vi "WCA_GET_AMC.vi"(0 "Cartridge Band":u32=10, 1 "Slave Node in":cluster{"Address":i16, "Serial Number":i8[]}={"Address"=19, "Serial Number"=[16, 71, 55, 76, 1, 8, 0, -15]} {"Serial Number" format="%.0x"; "Address" format="%.0x"}, 2 "ObjHandle in":u32, 11 "error in (no error)":errorcluster) -> (4 "ObjHandle out":u32=92930112, 8 "GET_AMC":T1={"AMC_A_DRAIN_V"=3.5023499, "AMC_A_DRAIN_C"=53.95508, "AMC_A_GATE_V"=-0.47195435, "AMC_B_DRAIN_V"=4.3559265, "AMC_B_DRAIN_C"=314.81934, "AMC_B_GATE_V"=-0.49163818, "AMC_E_DRAIN_V"=3.9920044, "AMC_E_DRAIN_C"=338.2721, "AMC_E_GATE_V"=-0.24505615, "AMC_3V_SUPPLY_V"=-13.493347, "AMC_5V_MON"=5.223694, "AMC_MULT_D_V"=0.0}, 15 "error out":errorcluster)   [LabVIEW 2017]
uses:
  WCA_Global.vi
panel:
  # "Vd [V]"
  # "Id [mA]"
  # "Vg [V]"
  # "AMC A"
  # "AMC B"
  # "AMC E"
  # "Node Address"
  # "Serial Number"
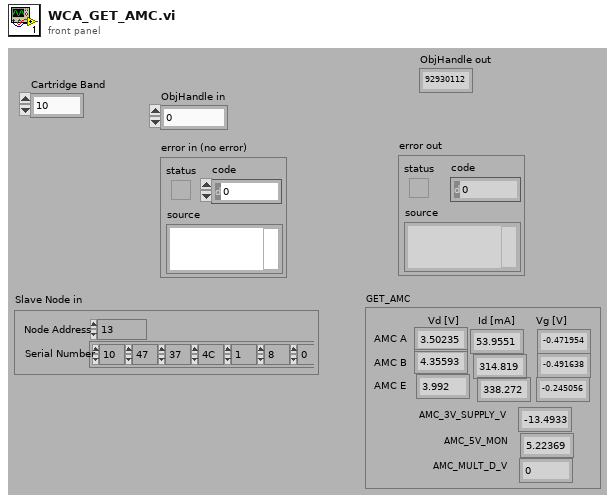
[diagram p1: front panel]
types:
  T1 = cluster{"AMC_A_DRAIN_V":sgl, "AMC_A_DRAIN_C":sgl, "AMC_A_GATE_V":sgl, "AMC_B_DRAIN_V":sgl, "AMC_B_DRAIN_C":sgl, "AMC_B_GATE_V":sgl, "AMC_E_DRAIN_V":sgl, "AMC_E_DRAIN_C":sgl, "AMC_E_GATE_V":sgl, "AMC_3V_SUPPLY_V":sgl, "AMC_5V_MON":sgl, "AMC_MULT_D_V":sgl}
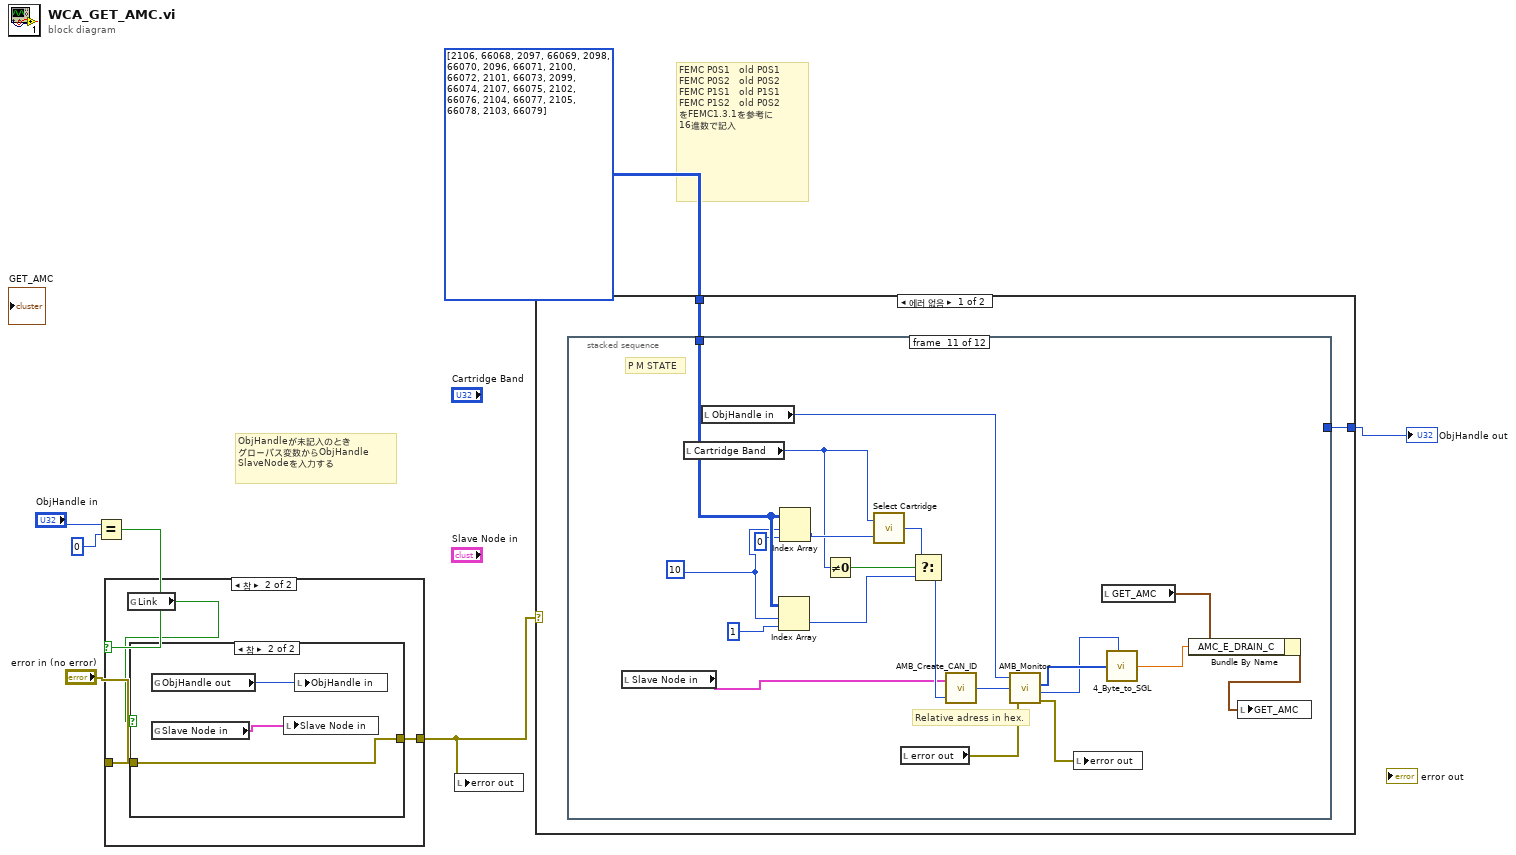
[diagram p0: block diagram]
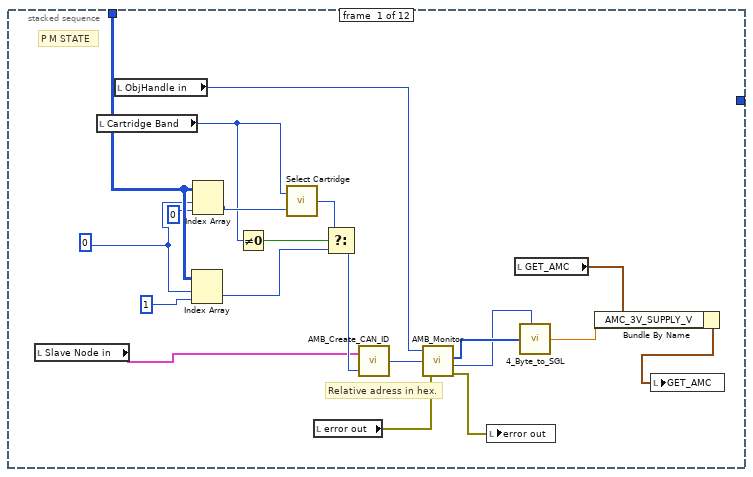
[diagram p2: hidden frame]
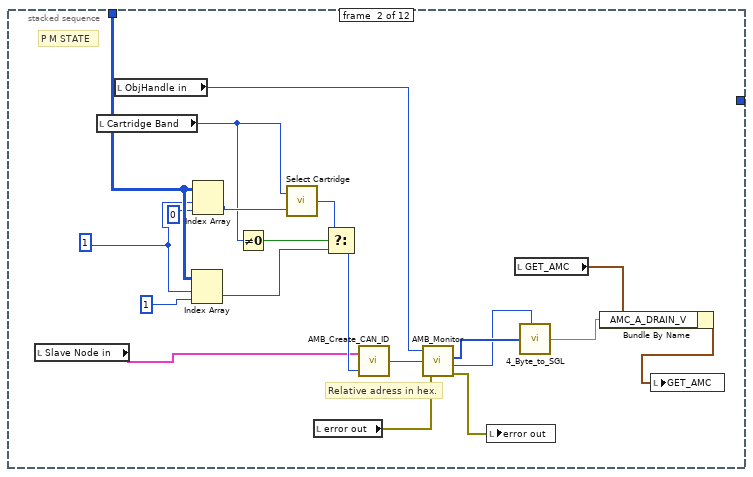
[diagram p3: hidden frame]
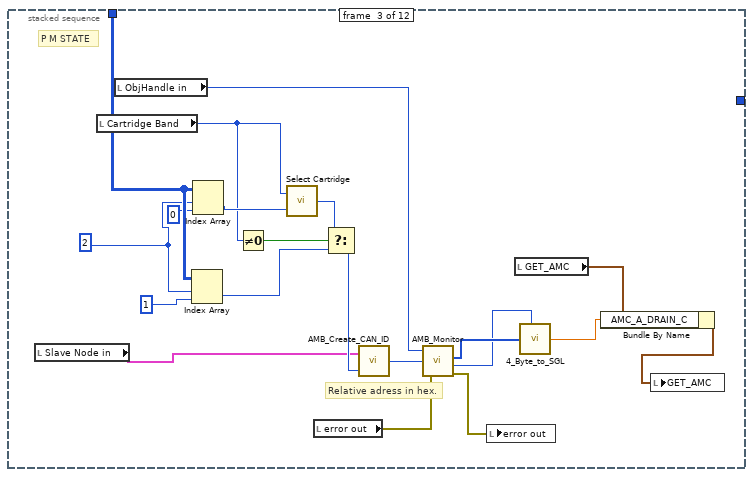
[diagram p4: hidden frame]
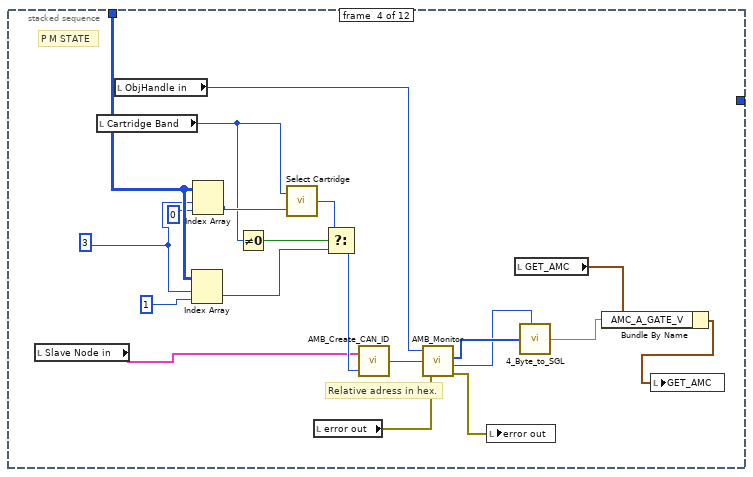
[diagram p5: hidden frame]
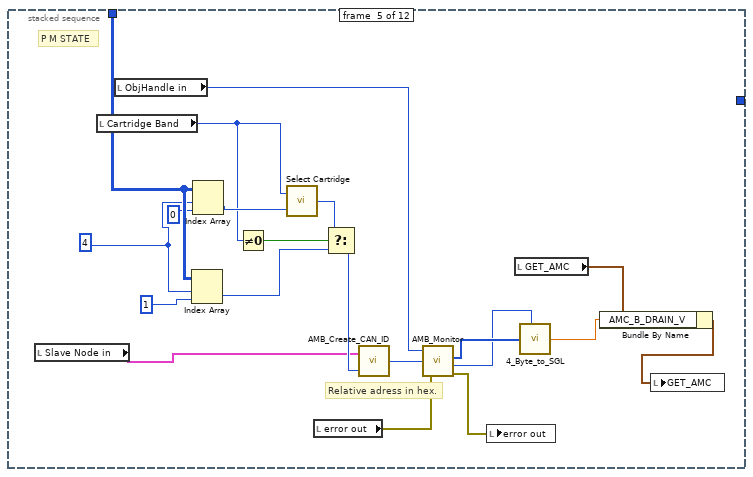
[diagram p6: hidden frame]
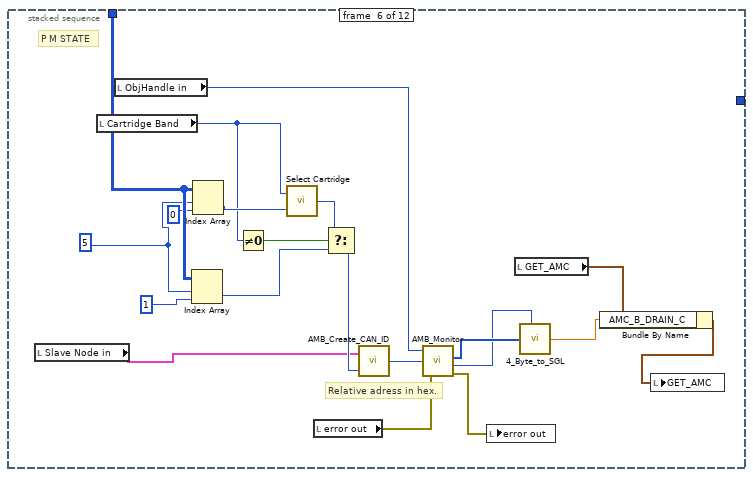
[diagram p7: hidden frame]
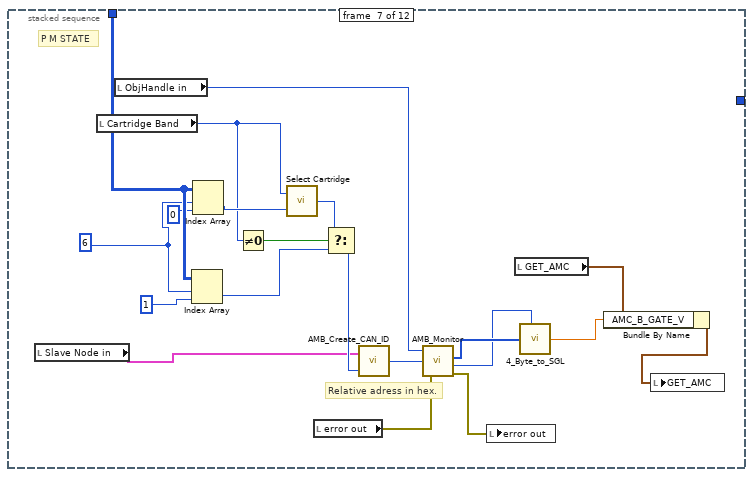
[diagram p8: hidden frame]
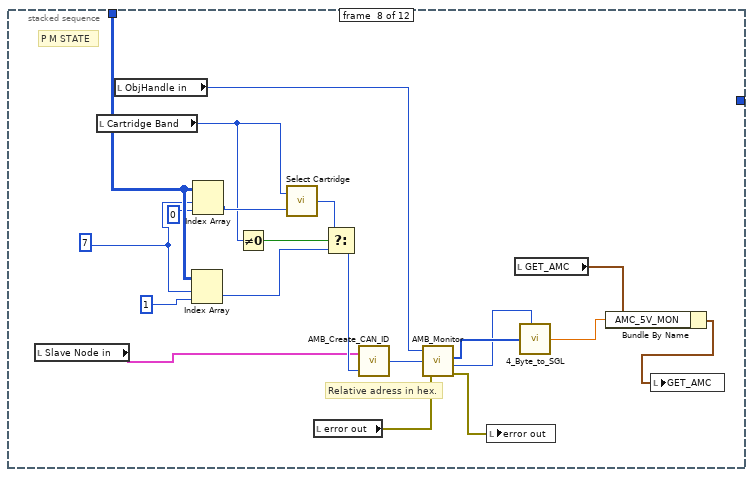
[diagram p9: hidden frame]
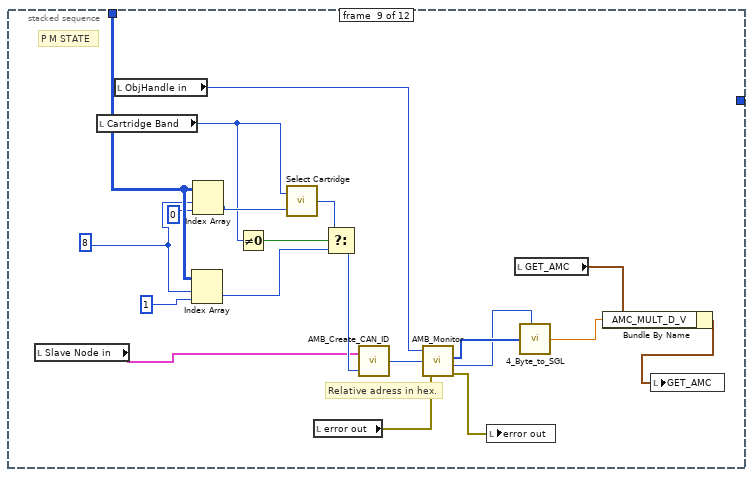
[diagram p10: hidden frame]
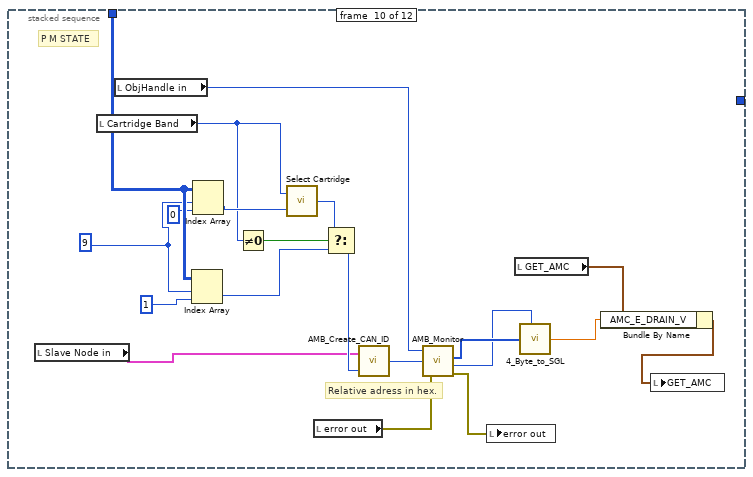
[diagram p11: hidden frame]
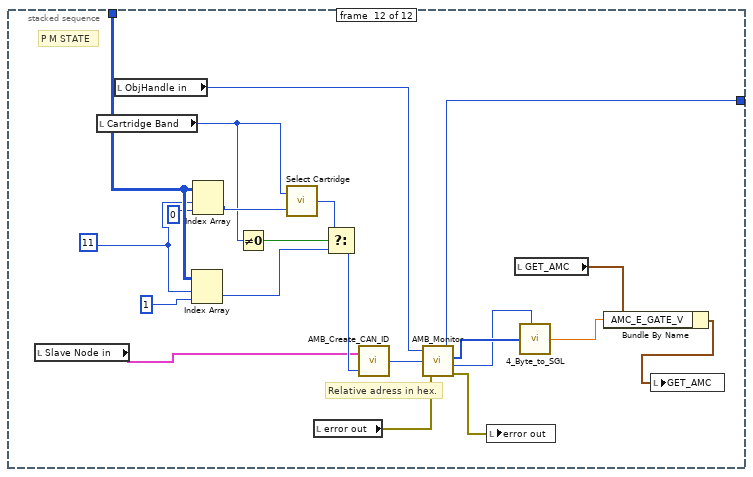
[diagram p12: hidden frame]
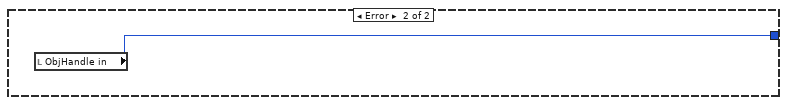
[diagram p13: hidden frame]
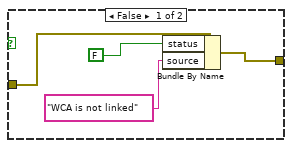
[diagram p15: hidden frame]
diagram:
  # "ObjHandleが未記入のとき\nグローバス変数からObjHandle\nSlaveNodeを入力する"
  # "FEMC P0S1   old P0S1\nFEMC P0S2   old P0S2\nFEMC P1S1   old P1S1\nFEMC P1S2   old P0S2\nをFEMC1.3.1を参考に\n16進数で記入"
  n1 = Equal?(x="ObjHandle in", y=0) -> (x = y?=w5:bool)
  n2 = case shown="참" w5 {
    tunnel: "error in (no error)" -> [w8 w11]
    tunnel: [w8 w10] -> w3
    frame False {
    }
    frame True {
      n3 = global read "WCA_Global.vi" "Link"() -> (w9:bool)
      n4 = case shown="참" w9 {
        tunnel: w11 -> [w15 w16]
        tunnel: [w12 w16] -> w10
        frame False {
          n5 = Bundle By Name(cluster=w15, "status"=FALSE, "source"="WCA is not linked") -> (w12:errorcluster)
        }
        frame True {
          n6 = global read "WCA_Global.vi" "ObjHandle out"() -> (w18:u32)
          n7 = global read "WCA_Global.vi" "Slave Node in"() -> (w17:cluster{"Address":i16, "Serial Number":i8[]})
          n8 = local write "Slave Node in"(w17) -> ()
          n9 = local write "ObjHandle in"(w18) -> ()
        }
      }
    }
  }
  n10 = local write "error out"(w3) -> ()
  n11 = case shown="에러 없음" w3 {
    tunnel: [w19 w262] -> w2
    tunnel: i32[][] [[2106, 66068], [2097, 66069], [2098, 66070], [2096, 66071], [2100, 66072], [2101, 66073], [2099, 66074], [2107, 66075], [2102, 66076], [2104, 66077], [2105, 66078], [2103, 66079]] -> [w20 _]
    frame No Error {
      n12 = stacked-sequence {
        tunnel: w20 -> [w40 w60 w80 w100 w120 w140 w160 w180 w200 w220 w240 w261]
        tunnel: [_ _ _ _ _ _ _ _ _ _ _ w241] -> w19
        frame #0 {
          w25 = 0
          # "Relative adress in hex."
          # "P M STATE"
          n13 = local read "Slave Node in"() -> (w24:cluster{"Address":i16, "Serial Number":i8[]})
          n14 = local read "Cartridge Band"() -> (w26:u32)
          n15 = local read "ObjHandle in"() -> (w36:u32)
          n16 = Index Array(array=w40, index (row)=w25, index (col)=1) -> (element=w35:i32)
          n17 = Index Array(array=w40, index (row)=w25, index (col)=0) -> (element=w34:i32)
          n18 = Not Equal To 0?(x=w26) -> (x != 0?=w37:bool)
          n19 = call "Select Cartridge.vi"("Relative Address in"=w34, "Cartridge band"=w26) -> ("Relative Address out"=w38:u32)
          n20 = local read "error out"() -> (w28:errorcluster)
          n21 = Select(t=w38, s=w37, f=w35) -> (s? t:f=w39:u32)
          n22 = call "AMB_Create_CAN_ID.vi"("Relative Address in"=w39, "Slave Node in"=w24) -> ("CAN ID out"=w31:u32)
          n23 = call "AMB_Monitor.vi"("ObjHandle in"=w36, "CAN ID in"=w31, "error in"=w28) -> ("Data Array out"=w23:u8[], "Data Length out"=w22:u8, "error out"=w27:errorcluster)  [unwired: 1 out]
          n24 = local write "error out"(w27) -> ()
          n25 = local read "GET_AMC"() -> (w30:T1)
          n26 = call "4_Byte_to_SGL.vi"("Array of 4 bytes"=w23, "number of valid bytes"=w22) -> ("Number"=w21:sgl)  [unwired: 1 out]
          n27 = Bundle By Name(cluster=w30, "AMC_3V_SUPPLY_V"=w21) -> (w29:T1)
          n28 = local write "GET_AMC"(w29) -> ()
        }
        frame #1 {
          w45 = 1
          # "Relative adress in hex."
          # "P M STATE"
          n29 = local read "Slave Node in"() -> (w44:cluster{"Address":i16, "Serial Number":i8[]})
          n30 = local read "Cartridge Band"() -> (w46:u32)
          n31 = local read "ObjHandle in"() -> (w56:u32)
          n32 = Index Array(array=w60, index (row)=w45, index (col)=1) -> (element=w55:i32)
          n33 = Index Array(array=w60, index (row)=w45, index (col)=0) -> (element=w54:i32)
          n34 = Not Equal To 0?(x=w46) -> (x != 0?=w57:bool)
          n35 = call "Select Cartridge.vi"("Relative Address in"=w54, "Cartridge band"=w46) -> ("Relative Address out"=w58:u32)
          n36 = local read "error out"() -> (w48:errorcluster)
          n37 = Select(t=w58, s=w57, f=w55) -> (s? t:f=w59:u32)
          n38 = call "AMB_Create_CAN_ID.vi"("Relative Address in"=w59, "Slave Node in"=w44) -> ("CAN ID out"=w51:u32)
          n39 = call "AMB_Monitor.vi"("ObjHandle in"=w56, "CAN ID in"=w51, "error in"=w48) -> ("Data Array out"=w43:u8[], "Data Length out"=w42:u8, "error out"=w47:errorcluster)  [unwired: 1 out]
          n40 = local write "error out"(w47) -> ()
          n41 = local read "GET_AMC"() -> (w50:T1)
          n42 = call "4_Byte_to_SGL.vi"("Array of 4 bytes"=w43, "number of valid bytes"=w42) -> ("Number"=w41:sgl)  [unwired: 1 out]
          n43 = Bundle By Name(cluster=w50, "AMC_A_DRAIN_V"=w41) -> (w49:T1)
          n44 = local write "GET_AMC"(w49) -> ()
        }
        frame #2 {
          w65 = 2
          # "Relative adress in hex."
          # "P M STATE"
          n45 = local read "Slave Node in"() -> (w64:cluster{"Address":i16, "Serial Number":i8[]})
          n46 = local read "Cartridge Band"() -> (w66:u32)
          n47 = local read "ObjHandle in"() -> (w76:u32)
          n48 = Index Array(array=w80, index (row)=w65, index (col)=1) -> (element=w75:i32)
          n49 = Index Array(array=w80, index (row)=w65, index (col)=0) -> (element=w74:i32)
          n50 = Not Equal To 0?(x=w66) -> (x != 0?=w77:bool)
          n51 = call "Select Cartridge.vi"("Relative Address in"=w74, "Cartridge band"=w66) -> ("Relative Address out"=w78:u32)
          n52 = local read "error out"() -> (w68:errorcluster)
          n53 = Select(t=w78, s=w77, f=w75) -> (s? t:f=w79:u32)
          n54 = call "AMB_Create_CAN_ID.vi"("Relative Address in"=w79, "Slave Node in"=w64) -> ("CAN ID out"=w71:u32)
          n55 = call "AMB_Monitor.vi"("ObjHandle in"=w76, "CAN ID in"=w71, "error in"=w68) -> ("Data Array out"=w63:u8[], "Data Length out"=w62:u8, "error out"=w67:errorcluster)  [unwired: 1 out]
          n56 = local write "error out"(w67) -> ()
          n57 = local read "GET_AMC"() -> (w70:T1)
          n58 = call "4_Byte_to_SGL.vi"("Array of 4 bytes"=w63, "number of valid bytes"=w62) -> ("Number"=w61:sgl)  [unwired: 1 out]
          n59 = Bundle By Name(cluster=w70, "AMC_A_DRAIN_C"=w61) -> (w69:T1)
          n60 = local write "GET_AMC"(w69) -> ()
        }
        frame #3 {
          w85 = 3
          # "Relative adress in hex."
          # "P M STATE"
          n61 = local read "Slave Node in"() -> (w84:cluster{"Address":i16, "Serial Number":i8[]})
          n62 = local read "Cartridge Band"() -> (w86:u32)
          n63 = local read "ObjHandle in"() -> (w96:u32)
          n64 = Index Array(array=w100, index (row)=w85, index (col)=1) -> (element=w95:i32)
          n65 = Index Array(array=w100, index (row)=w85, index (col)=0) -> (element=w94:i32)
          n66 = Not Equal To 0?(x=w86) -> (x != 0?=w97:bool)
          n67 = call "Select Cartridge.vi"("Relative Address in"=w94, "Cartridge band"=w86) -> ("Relative Address out"=w98:u32)
          n68 = local read "error out"() -> (w88:errorcluster)
          n69 = Select(t=w98, s=w97, f=w95) -> (s? t:f=w99:u32)
          n70 = call "AMB_Create_CAN_ID.vi"("Relative Address in"=w99, "Slave Node in"=w84) -> ("CAN ID out"=w91:u32)
          n71 = call "AMB_Monitor.vi"("ObjHandle in"=w96, "CAN ID in"=w91, "error in"=w88) -> ("Data Array out"=w83:u8[], "Data Length out"=w82:u8, "error out"=w87:errorcluster)  [unwired: 1 out]
          n72 = local write "error out"(w87) -> ()
          n73 = local read "GET_AMC"() -> (w90:T1)
          n74 = call "4_Byte_to_SGL.vi"("Array of 4 bytes"=w83, "number of valid bytes"=w82) -> ("Number"=w81:sgl)  [unwired: 1 out]
          n75 = Bundle By Name(cluster=w90, "AMC_A_GATE_V"=w81) -> (w89:T1)
          n76 = local write "GET_AMC"(w89) -> ()
        }
        frame #4 {
          w105 = 4
          # "Relative adress in hex."
          # "P M STATE"
          n77 = local read "Slave Node in"() -> (w104:cluster{"Address":i16, "Serial Number":i8[]})
          n78 = local read "Cartridge Band"() -> (w106:u32)
          n79 = local read "ObjHandle in"() -> (w116:u32)
          n80 = Index Array(array=w120, index (row)=w105, index (col)=1) -> (element=w115:i32)
          n81 = Index Array(array=w120, index (row)=w105, index (col)=0) -> (element=w114:i32)
          n82 = Not Equal To 0?(x=w106) -> (x != 0?=w117:bool)
          n83 = call "Select Cartridge.vi"("Relative Address in"=w114, "Cartridge band"=w106) -> ("Relative Address out"=w118:u32)
          n84 = local read "error out"() -> (w108:errorcluster)
          n85 = Select(t=w118, s=w117, f=w115) -> (s? t:f=w119:u32)
          n86 = call "AMB_Create_CAN_ID.vi"("Relative Address in"=w119, "Slave Node in"=w104) -> ("CAN ID out"=w111:u32)
          n87 = call "AMB_Monitor.vi"("ObjHandle in"=w116, "CAN ID in"=w111, "error in"=w108) -> ("Data Array out"=w103:u8[], "Data Length out"=w102:u8, "error out"=w107:errorcluster)  [unwired: 1 out]
          n88 = local write "error out"(w107) -> ()
          n89 = local read "GET_AMC"() -> (w110:T1)
          n90 = call "4_Byte_to_SGL.vi"("Array of 4 bytes"=w103, "number of valid bytes"=w102) -> ("Number"=w101:sgl)  [unwired: 1 out]
          n91 = Bundle By Name(cluster=w110, "AMC_B_DRAIN_V"=w101) -> (w109:T1)
          n92 = local write "GET_AMC"(w109) -> ()
        }
        frame #5 {
          w125 = 5
          # "Relative adress in hex."
          # "P M STATE"
          n93 = local read "Slave Node in"() -> (w124:cluster{"Address":i16, "Serial Number":i8[]})
          n94 = local read "Cartridge Band"() -> (w126:u32)
          n95 = local read "ObjHandle in"() -> (w136:u32)
          n96 = Index Array(array=w140, index (row)=w125, index (col)=1) -> (element=w135:i32)
          n97 = Index Array(array=w140, index (row)=w125, index (col)=0) -> (element=w134:i32)
          n98 = Not Equal To 0?(x=w126) -> (x != 0?=w137:bool)
          n99 = call "Select Cartridge.vi"("Relative Address in"=w134, "Cartridge band"=w126) -> ("Relative Address out"=w138:u32)
          n100 = local read "error out"() -> (w128:errorcluster)
          n101 = Select(t=w138, s=w137, f=w135) -> (s? t:f=w139:u32)
          n102 = call "AMB_Create_CAN_ID.vi"("Relative Address in"=w139, "Slave Node in"=w124) -> ("CAN ID out"=w131:u32)
          n103 = call "AMB_Monitor.vi"("ObjHandle in"=w136, "CAN ID in"=w131, "error in"=w128) -> ("Data Array out"=w123:u8[], "Data Length out"=w122:u8, "error out"=w127:errorcluster)  [unwired: 1 out]
          n104 = local write "error out"(w127) -> ()
          n105 = local read "GET_AMC"() -> (w130:T1)
          n106 = call "4_Byte_to_SGL.vi"("Array of 4 bytes"=w123, "number of valid bytes"=w122) -> ("Number"=w121:sgl)  [unwired: 1 out]
          n107 = Bundle By Name(cluster=w130, "AMC_B_DRAIN_C"=w121) -> (w129:T1)
          n108 = local write "GET_AMC"(w129) -> ()
        }
        frame #6 {
          w145 = 6
          # "Relative adress in hex."
          # "P M STATE"
          n109 = local read "Slave Node in"() -> (w144:cluster{"Address":i16, "Serial Number":i8[]})
          n110 = local read "Cartridge Band"() -> (w146:u32)
          n111 = local read "ObjHandle in"() -> (w156:u32)
          n112 = Index Array(array=w160, index (row)=w145, index (col)=1) -> (element=w155:i32)
          n113 = Index Array(array=w160, index (row)=w145, index (col)=0) -> (element=w154:i32)
          n114 = Not Equal To 0?(x=w146) -> (x != 0?=w157:bool)
          n115 = call "Select Cartridge.vi"("Relative Address in"=w154, "Cartridge band"=w146) -> ("Relative Address out"=w158:u32)
          n116 = local read "error out"() -> (w148:errorcluster)
          n117 = Select(t=w158, s=w157, f=w155) -> (s? t:f=w159:u32)
          n118 = call "AMB_Create_CAN_ID.vi"("Relative Address in"=w159, "Slave Node in"=w144) -> ("CAN ID out"=w151:u32)
          n119 = call "AMB_Monitor.vi"("ObjHandle in"=w156, "CAN ID in"=w151, "error in"=w148) -> ("Data Array out"=w143:u8[], "Data Length out"=w142:u8, "error out"=w147:errorcluster)  [unwired: 1 out]
          n120 = local write "error out"(w147) -> ()
          n121 = local read "GET_AMC"() -> (w150:T1)
          n122 = call "4_Byte_to_SGL.vi"("Array of 4 bytes"=w143, "number of valid bytes"=w142) -> ("Number"=w141:sgl)  [unwired: 1 out]
          n123 = Bundle By Name(cluster=w150, "AMC_B_GATE_V"=w141) -> (w149:T1)
          n124 = local write "GET_AMC"(w149) -> ()
        }
        frame #7 {
          w165 = 7
          # "Relative adress in hex."
          # "P M STATE"
          n125 = local read "Slave Node in"() -> (w164:cluster{"Address":i16, "Serial Number":i8[]})
          n126 = local read "Cartridge Band"() -> (w166:u32)
          n127 = local read "ObjHandle in"() -> (w176:u32)
          n128 = Index Array(array=w180, index (row)=w165, index (col)=1) -> (element=w175:i32)
          n129 = Index Array(array=w180, index (row)=w165, index (col)=0) -> (element=w174:i32)
          n130 = Not Equal To 0?(x=w166) -> (x != 0?=w177:bool)
          n131 = call "Select Cartridge.vi"("Relative Address in"=w174, "Cartridge band"=w166) -> ("Relative Address out"=w178:u32)
          n132 = local read "error out"() -> (w168:errorcluster)
          n133 = Select(t=w178, s=w177, f=w175) -> (s? t:f=w179:u32)
          n134 = call "AMB_Create_CAN_ID.vi"("Relative Address in"=w179, "Slave Node in"=w164) -> ("CAN ID out"=w171:u32)
          n135 = call "AMB_Monitor.vi"("ObjHandle in"=w176, "CAN ID in"=w171, "error in"=w168) -> ("Data Array out"=w163:u8[], "Data Length out"=w162:u8, "error out"=w167:errorcluster)  [unwired: 1 out]
          n136 = local write "error out"(w167) -> ()
          n137 = local read "GET_AMC"() -> (w170:T1)
          n138 = call "4_Byte_to_SGL.vi"("Array of 4 bytes"=w163, "number of valid bytes"=w162) -> ("Number"=w161:sgl)  [unwired: 1 out]
          n139 = Bundle By Name(cluster=w170, "AMC_5V_MON"=w161) -> (w169:T1)
          n140 = local write "GET_AMC"(w169) -> ()
        }
        frame #8 {
          w185 = 8
          # "Relative adress in hex."
          # "P M STATE"
          n141 = local read "Slave Node in"() -> (w184:cluster{"Address":i16, "Serial Number":i8[]})
          n142 = local read "Cartridge Band"() -> (w186:u32)
          n143 = local read "ObjHandle in"() -> (w196:u32)
          n144 = Index Array(array=w200, index (row)=w185, index (col)=1) -> (element=w195:i32)
          n145 = Index Array(array=w200, index (row)=w185, index (col)=0) -> (element=w194:i32)
          n146 = Not Equal To 0?(x=w186) -> (x != 0?=w197:bool)
          n147 = call "Select Cartridge.vi"("Relative Address in"=w194, "Cartridge band"=w186) -> ("Relative Address out"=w198:u32)
          n148 = local read "error out"() -> (w188:errorcluster)
          n149 = Select(t=w198, s=w197, f=w195) -> (s? t:f=w199:u32)
          n150 = call "AMB_Create_CAN_ID.vi"("Relative Address in"=w199, "Slave Node in"=w184) -> ("CAN ID out"=w191:u32)
          n151 = call "AMB_Monitor.vi"("ObjHandle in"=w196, "CAN ID in"=w191, "error in"=w188) -> ("Data Array out"=w183:u8[], "Data Length out"=w182:u8, "error out"=w187:errorcluster)  [unwired: 1 out]
          n152 = local write "error out"(w187) -> ()
          n153 = local read "GET_AMC"() -> (w190:T1)
          n154 = call "4_Byte_to_SGL.vi"("Array of 4 bytes"=w183, "number of valid bytes"=w182) -> ("Number"=w181:sgl)  [unwired: 1 out]
          n155 = Bundle By Name(cluster=w190, "AMC_MULT_D_V"=w181) -> (w189:T1)
          n156 = local write "GET_AMC"(w189) -> ()
        }
        frame #9 {
          w205 = 9
          # "Relative adress in hex."
          # "P M STATE"
          n157 = local read "Slave Node in"() -> (w204:cluster{"Address":i16, "Serial Number":i8[]})
          n158 = local read "Cartridge Band"() -> (w206:u32)
          n159 = local read "ObjHandle in"() -> (w216:u32)
          n160 = Index Array(array=w220, index (row)=w205, index (col)=1) -> (element=w215:i32)
          n161 = Index Array(array=w220, index (row)=w205, index (col)=0) -> (element=w214:i32)
          n162 = Not Equal To 0?(x=w206) -> (x != 0?=w217:bool)
          n163 = call "Select Cartridge.vi"("Relative Address in"=w214, "Cartridge band"=w206) -> ("Relative Address out"=w218:u32)
          n164 = local read "error out"() -> (w208:errorcluster)
          n165 = Select(t=w218, s=w217, f=w215) -> (s? t:f=w219:u32)
          n166 = call "AMB_Create_CAN_ID.vi"("Relative Address in"=w219, "Slave Node in"=w204) -> ("CAN ID out"=w211:u32)
          n167 = call "AMB_Monitor.vi"("ObjHandle in"=w216, "CAN ID in"=w211, "error in"=w208) -> ("Data Array out"=w203:u8[], "Data Length out"=w202:u8, "error out"=w207:errorcluster)  [unwired: 1 out]
          n168 = local write "error out"(w207) -> ()
          n169 = local read "GET_AMC"() -> (w210:T1)
          n170 = call "4_Byte_to_SGL.vi"("Array of 4 bytes"=w203, "number of valid bytes"=w202) -> ("Number"=w201:sgl)  [unwired: 1 out]
          n171 = Bundle By Name(cluster=w210, "AMC_E_DRAIN_V"=w201) -> (w209:T1)
          n172 = local write "GET_AMC"(w209) -> ()
        }
        frame #10 {
          w225 = 10
          # "Relative adress in hex."
          # "P M STATE"
          n173 = local read "Slave Node in"() -> (w224:cluster{"Address":i16, "Serial Number":i8[]})
          n174 = local read "Cartridge Band"() -> (w226:u32)
          n175 = local read "ObjHandle in"() -> (w236:u32)
          n176 = Index Array(array=w240, index (row)=w225, index (col)=1) -> (element=w235:i32)
          n177 = Index Array(array=w240, index (row)=w225, index (col)=0) -> (element=w234:i32)
          n178 = Not Equal To 0?(x=w226) -> (x != 0?=w237:bool)
          n179 = call "Select Cartridge.vi"("Relative Address in"=w234, "Cartridge band"=w226) -> ("Relative Address out"=w238:u32)
          n180 = local read "error out"() -> (w228:errorcluster)
          n181 = Select(t=w238, s=w237, f=w235) -> (s? t:f=w239:u32)
          n182 = call "AMB_Create_CAN_ID.vi"("Relative Address in"=w239, "Slave Node in"=w224) -> ("CAN ID out"=w231:u32)
          n183 = call "AMB_Monitor.vi"("ObjHandle in"=w236, "CAN ID in"=w231, "error in"=w228) -> ("Data Array out"=w223:u8[], "Data Length out"=w222:u8, "error out"=w227:errorcluster)  [unwired: 1 out]
          n184 = local write "error out"(w227) -> ()
          n185 = local read "GET_AMC"() -> (w230:T1)
          n186 = call "4_Byte_to_SGL.vi"("Array of 4 bytes"=w223, "number of valid bytes"=w222) -> ("Number"=w221:sgl)  [unwired: 1 out]
          n187 = Bundle By Name(cluster=w230, "AMC_E_DRAIN_C"=w221) -> (w229:T1)
          n188 = local write "GET_AMC"(w229) -> ()
        }
        frame #11 {
          w246 = 11
          # "Relative adress in hex."
          # "P M STATE"
          n189 = local read "Slave Node in"() -> (w245:cluster{"Address":i16, "Serial Number":i8[]})
          n190 = local read "Cartridge Band"() -> (w247:u32)
          n191 = local read "ObjHandle in"() -> (w257:u32)
          n192 = Index Array(array=w261, index (row)=w246, index (col)=1) -> (element=w256:i32)
          n193 = Index Array(array=w261, index (row)=w246, index (col)=0) -> (element=w255:i32)
          n194 = Not Equal To 0?(x=w247) -> (x != 0?=w258:bool)
          n195 = call "Select Cartridge.vi"("Relative Address in"=w255, "Cartridge band"=w247) -> ("Relative Address out"=w259:u32)
          n196 = local read "error out"() -> (w249:errorcluster)
          n197 = Select(t=w259, s=w258, f=w256) -> (s? t:f=w260:u32)
          n198 = call "AMB_Create_CAN_ID.vi"("Relative Address in"=w260, "Slave Node in"=w245) -> ("CAN ID out"=w252:u32)
          n199 = call "AMB_Monitor.vi"("ObjHandle in"=w257, "CAN ID in"=w252, "error in"=w249) -> ("ObjHandle out"=w241:u32, "Data Array out"=w244:u8[], "Data Length out"=w243:u8, "error out"=w248:errorcluster)
          n200 = local write "error out"(w248) -> ()
          n201 = local read "GET_AMC"() -> (w251:T1)
          n202 = call "4_Byte_to_SGL.vi"("Array of 4 bytes"=w244, "number of valid bytes"=w243) -> ("Number"=w242:sgl)  [unwired: 1 out]
          n203 = Bundle By Name(cluster=w251, "AMC_E_GATE_V"=w242) -> (w250:T1)
          n204 = local write "GET_AMC"(w250) -> ()
        }
      }
    }
    frame Error {
      n205 = local read "ObjHandle in"() -> (w262:u32)
    }
  }
  "ObjHandle out" <- w2
